vi "Cannon Lock Fire.vi"(1 "Cannon Info In":T2) -> (0 "Cannon Info Out":T2)   [LabVIEW 2013]
uses:
  <vilib>/Rock Robotics/WPI/Relay/WPI_RelayValue.ctl
  <vilib>/Rock Robotics/WPI/Solenoid/WPI_SolenoidValue.ctl
  Intake/Intake Global.vi
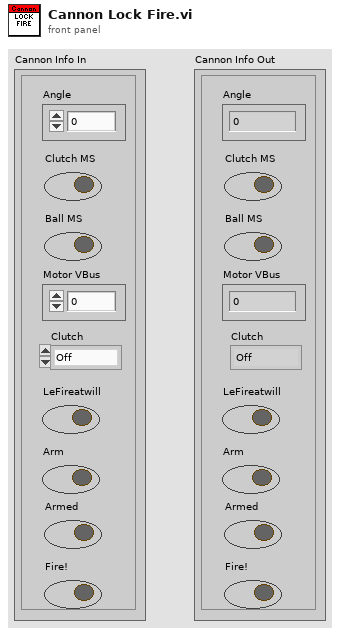
[diagram p1: front panel]
types:
  T1 = typedef "WPI_RelayValue.ctl" = enum16{"Off", "On", "Forward", "Reverse"}
  T2 = cluster{"Angle":dbl, "Clutch MS":bool, "Ball MS":bool, "Motor VBus":dbl, "Clutch ":T1, "LeFireatwill":bool, "Arm":bool, "Armed":bool, "Fire!":bool}
  T3 = typedef "WPI_SolenoidValue.ctl" = enum16{"Off", "On", "Forward", "Reverse"}
  T4 = cluster{"Arm State":bool, "Gripper In":bool, "Gripper Out":bool, "Gripper Execution":T1, "Arm Execution":T3, "Middle MS":bool, "Middle Stop":bool}
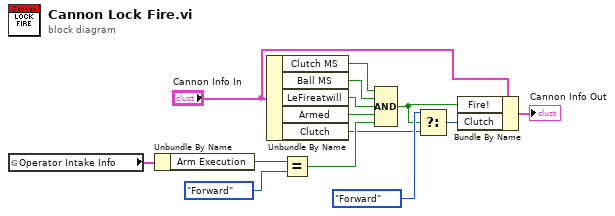
[diagram p0: block diagram]
diagram:
  n1 = global read "Intake Global.vi" "Operator Intake Info"() -> (w8:T4)
  n2 = Unbundle By Name(w8) -> ("Arm Execution"=w7:T3)
  n3 = Unbundle By Name("Cannon Info In") -> ("Clutch MS"=w9:bool, "Ball MS"=w10:bool, "LeFireatwill"=w12:bool, "Armed"=w11:bool, "Clutch"=w2:T1)
  n4 = Equal?(x=w7, y=WPI_SolenoidValue."Forward" ("Arm Execution")) -> (x = y?=w5:bool)
  n5 = Compound Arithmetic op=AND(w9, w10, w12, w11, w5) -> (w1:bool)
  n6 = Select(t=WPI_SolenoidValue."Forward" ("Arm Execution"), s=w1, f=w2) -> (s? t:f=w4:T1)
  n7 = Bundle By Name(cluster="Cannon Info In", "Fire!"=w1, "Clutch"=w4) -> (→"Cannon Info Out":T2)
